vi "Start.vi"(6 "Mode":T1, 7 "[x]":T2, 8 "error in (no error)":errorcluster, 11 "Serial Port in":refnum<visa-resource-name>) -> (0 "error out":errorcluster, 3 "Serial Port out":refnum<visa-resource-name>)   [LabVIEW 2022 SP3, in "Chemyx_Syringe_Pump_driver.lvlib"]
doc: "Starts the operation of the pump using the parameters currently loaded into the pump."
uses:
  Chemyx_Syringe_Pump_driver.lvlib
  _private/Control/Control Mode.ctl
  _private/Control/Programmable Mode.ctl
panel:
  # "Starts the operation of the pump using the parameters currently loaded into the pump."
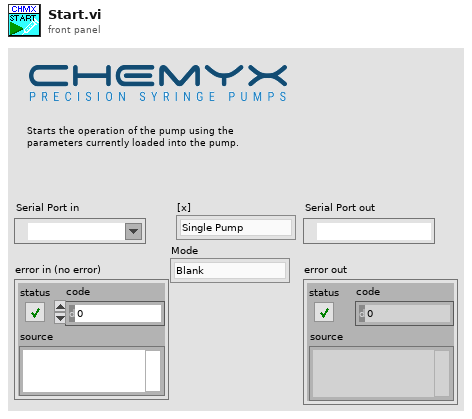
[diagram p1: front panel]
types:
  T1 = typedef "Chemyx_Syringe_Pump_driver.lvlib/Programmable Mode.ctl" = enum16{"Blank", "Basic", "Programmable"}
  T2 = typedef "Chemyx_Syringe_Pump_driver.lvlib/Control Mode.ctl" = enum16{"Single Pump", "Pump Channel 1", "Pump Channel 2", "Cycle Mode"}
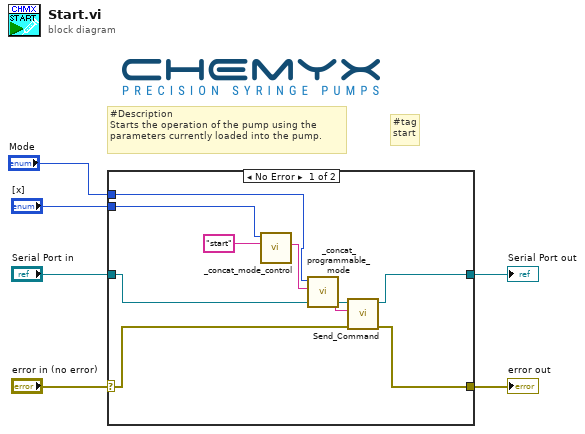
[diagram p0: block diagram]
diagram:
  # "#tag\nstart"
  # "#Description\nStarts the operation of the pump using the parameters currently loaded into the pump."
  n1 = case shown="No Error" "error in (no error)" {
    selector: "error in (no error)" -> [w14 w17]
    tunnel: "Serial Port in" -> [w15 w16]
    tunnel: [w13 w17] -> w4
    tunnel: [w12 w16] -> w3
    tunnel: "[x]" -> [w10 _]
    tunnel: "Mode" -> [w7 _]
    frame No Error {
      n2 = call "_concat_mode_control.vi"("write buffer"="start", "[x]"=w10) -> ("write buffer out"=w9:string)  [unwired: 9 in]
      n3 = call "_concat_programmable_mode.vi"("write buffer"=w9, "Programmable Mode"=w7) -> ("write buffer out"=w8:string)  [unwired: 9 in]
      n4 = call "Send_Command.vi"("error in (no error)"=w14, "write buffer"=w8, "Serial Port in"=w15) -> ("error out"=w13:errorcluster, "VISA Refnum out"=w12:refnum<visa-resource-name>)  [unwired: 6 in, 1 out]
    }
    frame Error {
    }
  }
  "error out" <- w4
  "Serial Port out" <- w3
